vi "Server.vi"() -> ()   [LabVIEW 2024]
uses:
  <vilib>/Utility/file.llb/Read Delimited Spreadsheet (string).vi
  <vilib>/Utility/file.llb/Write Delimited Spreadsheet (string).vi
panel:
  in  "BTN Refresh":bool
  in  "Member":string[][](table)
  in  "Car Wash Record":string[][](table)
  # "Car Wash Record"
  # "Registered Member"
  # "Refresh"
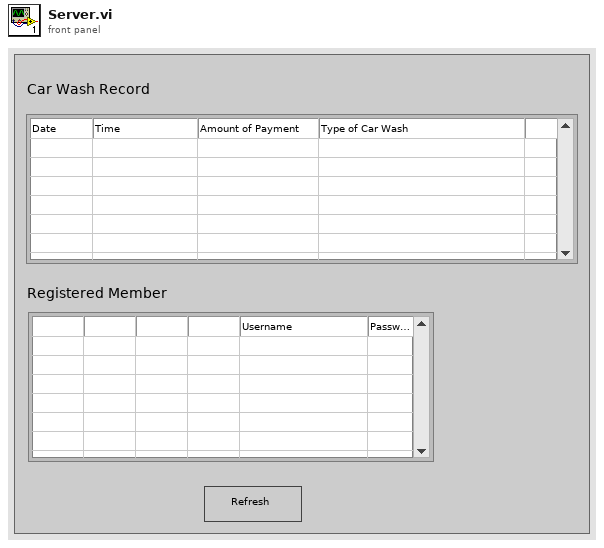
[diagram p1: front panel]
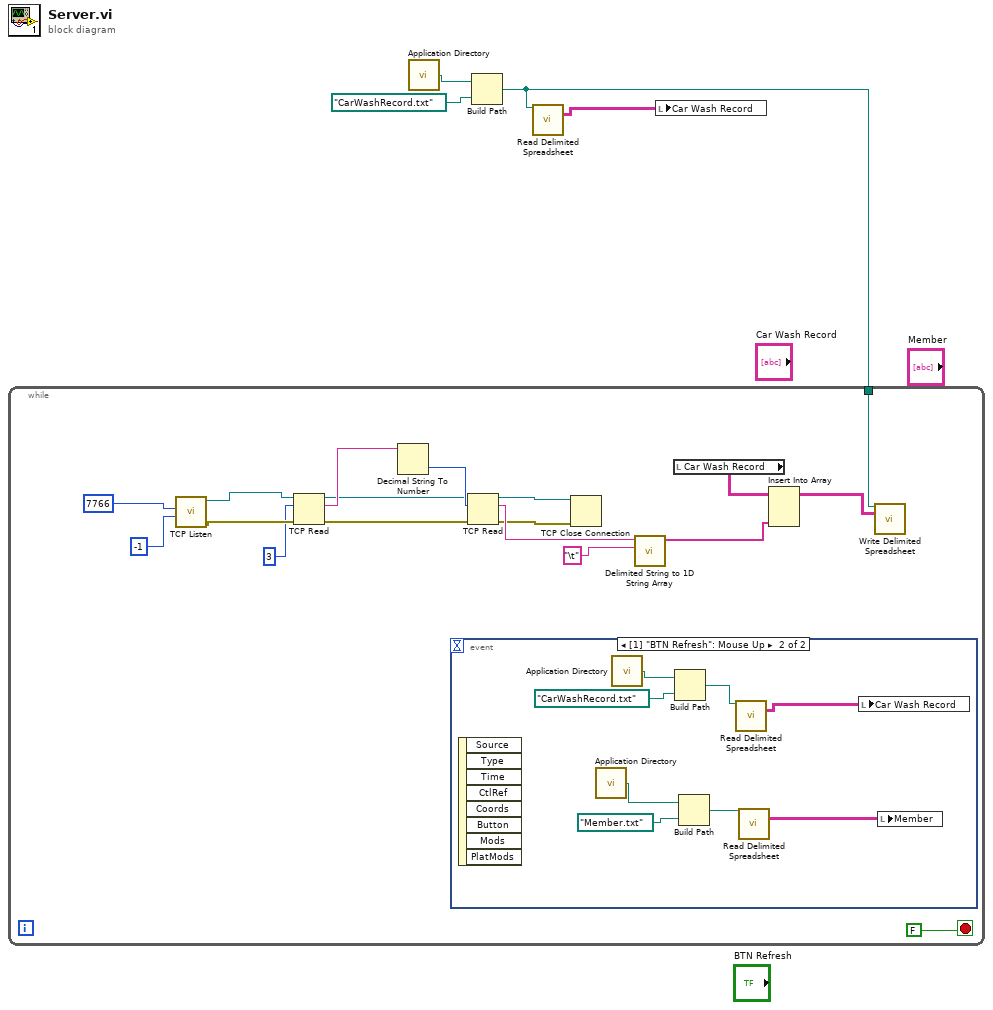
[diagram p0: block diagram]
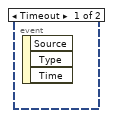
[diagram p2: hidden frame]
diagram:
  n1 = call <vilib>:"Application Directory.vi"() -> ("Application Directory"=w3:path)
  n2 = Build Path(base path=w3, name or relative path=path "CarWashRecord.txt") -> (appended path=w1:path)
  n3 = while {
    tunnel: w1 -> [w9]
    stop <- FALSE stop-if-true
    n4 = call <vilib>:"TCP Listen.vi"("timeout ms (wait forever: -1)"=-1, "port"=u16 7766) -> ("error out"=w17:errorcluster, "connection ID"=w18:refnum<k5>)  [unwired: 5 in, 3 out]
    n5 = TCP Read(connection ID=w18, bytes to read=3 ("timeout ms (25000)"), error in (no error)=w17) -> (connection ID out=w10:refnum<k5>, data out=w14:string, error out=w11:errorcluster)  [unwired: 2 in]
    n6 = Decimal String To Number(string=w14) -> (number=w15:i32)  [unwired: 2 in, 1 out]
    n7 = event shown="[1] \"BTN Refresh\": Mouse Up" {
      selector: _ -> [_ _]
      dyn-events: _ -> [_ _]
      timeout: _ -> [_ _]
      event Timeout {
        n8 = event-data() -> ()  [unwired: 1 in, 3 out]
      }
      event "BTN Refresh": Mouse Up {
        n9 = event-data() -> ()  [unwired: 1 in, 8 out]
        n10 = call <vilib>:"Application Directory.vi"() -> ("Application Directory"=w23:path)
        n11 = call <vilib>:"Application Directory.vi"() -> ("Application Directory"=w28:path)
        n12 = Build Path(base path=w28, name or relative path=path "CarWashRecord.txt") -> (appended path=w30:path)
        n13 = Build Path(base path=w23, name or relative path=path "Member.txt") -> (appended path=w27:path)
        n14 = call-poly <vilib>:"Read Delimited Spreadsheet.vi"("file path (dialog if empty)"=w30) -> ("all rows"=w29:string[][])  [unwired: 9 in, 5 out]
        n15 = call-poly <vilib>:"Read Delimited Spreadsheet.vi"("file path (dialog if empty)"=w27) -> ("all rows"=w24:string[][])  [unwired: 9 in, 5 out]
        n16 = local write "Car Wash Record"(w29) -> ()
        n17 = local write "Member"(w24) -> ()
      }
    }
    n18 = TCP Read(connection ID=w10, bytes to read=w15, error in (no error)=w11) -> (connection ID out=w12:refnum<k5>, data out=w16:string, error out=w13:errorcluster)  [unwired: 2 in]
    n19 = TCP Close Connection(connection ID=w12, error in (no error)=w13) -> ()  [unwired: 1 in, 2 out]
    n20 = call <vilib>:"Delimited String to 1D String Array.vi"("delimiter"="\t", "delimited string"=w16) -> ("string array"=w19:string[])  [unwired: 9 in]
    n21 = local read "Car Wash Record"() -> (w20:string[][])
    n22 = Insert Into Array(array=w20, new element=w19) -> (w21:string[][])  [unwired: 2 in]
    n23 = call-poly <vilib>:"Write Delimited Spreadsheet.vi"("file path (dialog if empty)"=w9, "2D data"=w21) -> ()  [unwired: 12 in, 2 out]
  }
  n24 = call-poly <vilib>:"Read Delimited Spreadsheet.vi"("file path (dialog if empty)"=w1) -> ("all rows"=w2:string[][])  [unwired: 9 in, 5 out]
  n25 = local write "Car Wash Record"(w2) -> ()
